vi "Test Config Iface Readback U32.vi"(8 "error in (no error)":errorcluster, 11 "Test Case In":refnum<class "Configuration Interface Test.lvclass">) -> (0 "error out":errorcluster, 3 "Test Case Out":refnum<class "Configuration Interface Test.lvclass">)   [LabVIEW 2020, in "Configuration Interface Test.lvclass"]
uses:
  Configuration Interface Test.lvclass
  C:/Program Files (x86)/National Instruments/LabVIEW 2020/vi.lib/Asteme/LUnit/Test Case.lvclass
  Framework/Configuration/Configuration.lvclass
  <vilib>/Asteme/LUnit/Test Case.lvclass/Test Case.ctl
  <vilib>/Asteme/LUnit/LUnit Assertion Result.lvclass/LUnit Assertion Result.ctl
  <vilib>/Asteme/LUnit/Palette/Pass.vi
  <vilib>/Asteme/LUnit/Palette/Fail.vi
  <vilib>/Asteme/LUnit/Variant to string.vi
  <vilib>/Asteme/LUnit/Set Assertion Type.vi
  <vilib>/Asteme/LUnit/Add test result.vi
  <vilib>/Asteme/LUnit/LUnit Get Test Case.vi
  <vilib>/Asteme/LUnit/Assertion Result/LUnit Get Test Name.vi
  <vilib>/Asteme/LUnit/LUnit Write Message.vi
  <vilib>/Asteme/LUnit/LUnit Write Description.vi
  <vilib>/Asteme/LUnit/LUnit Write Skipped.vi
  <vilib>/Asteme/LUnit/LUnit Write Passed.vi
  <vilib>/Asteme/LUnit/LUnit Write Assertion Type.vi
  <vilib>/Asteme/LUnit/Read Test Case Name.vi
  <vilib>/Utility/Data Type/Get Type Information.vi
  <vilib>/Utility/LVClass/Get LV Class Name.vi
  <vilib>/Asteme/LUnit/LUnit Assertion Result.lvclass
  <vilib>/Asteme/LUnit/Test Case.lvclass
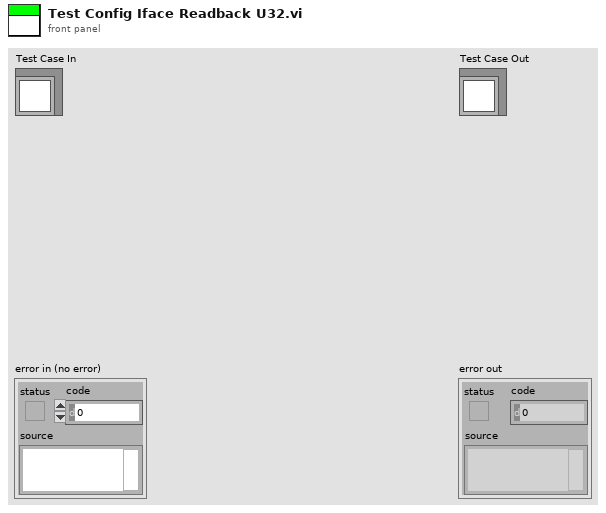
[diagram p1: front panel]
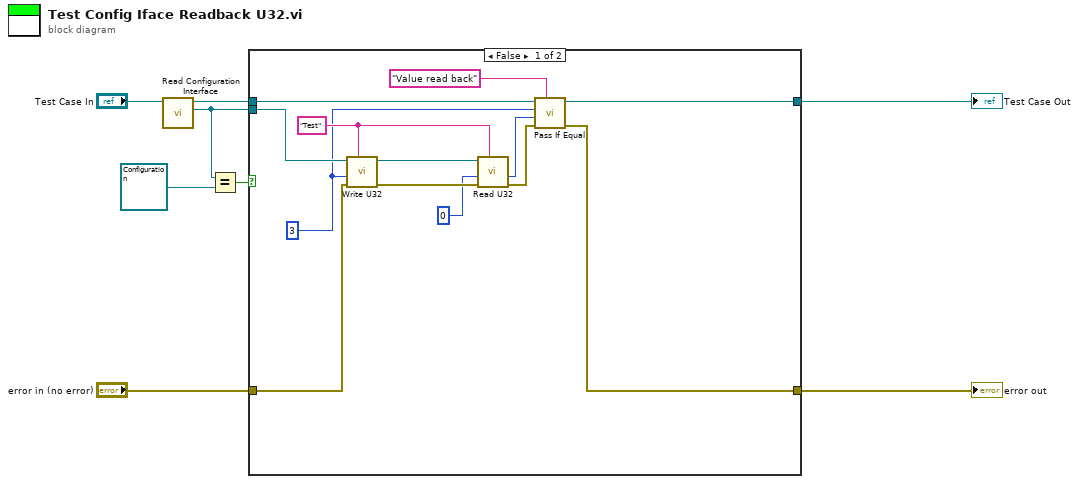
[diagram p0: block diagram]
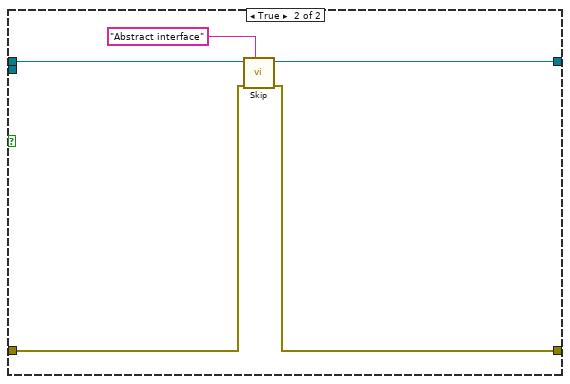
[diagram p2: hidden frame]
diagram:
  n1 = call "Read Configuration Interface.vi"("Configuration Interface Test In"="Test Case In") -> ("Configuration"=w3:refnum<class "Configuration.lvclass">, "Configuration Interface Test Out"=w6:refnum<class "Configuration Interface Test.lvclass">)  [unwired: 9 in]
  n2 = Equal?(x=w3, y=refnum<class "Configuration.lvclass"> refnum ("Configuration")) -> (x = y?=w1:bool)
  n3 = case shown="False" w1 {
    tunnel: [w18 w23] -> w7
    tunnel: w6 -> [w17 w26]
    tunnel: [w16 w25] -> w5
    tunnel: "error in (no error)" -> [w11 w24]
    tunnel: w3 -> [w14 _]
    frame False {
      w10 = u32 3
      w19 = "Test" ("key")
      n4 = call-dynamic "Write U32.vi"("key"=w19, "error in (no error)"=w11, "Value"=w10, "Configuration File In"=w14) -> ("error out"=w20:errorcluster, "Configuration File Out"=w21:refnum<class "Configuration.lvclass">)  [unwired: 6 in]
      n5 = call-dynamic "Read U32.vi"("key"=w19, "error in (no error)"=w20, "default value"=u32 0, "Configuration File In"=w21) -> ("error out"=w15:errorcluster, "value"=w12:u32)  [unwired: 5 in, 1 out]
      n6 = call <vilib>:"Pass If Equal.vi"("Description"="Value read back", "error in (no error)"=w15, "Actual"=w12, "Expected"=w10, "Test Case In"=w17) -> ("error out"=w18:errorcluster, "Test Case Out"=w16:refnum<class "Configuration Interface Test.lvclass">)  [unwired: 5 in]
    }
    frame True {
      n7 = call <vilib>:"Skip.vi"("Description"="Abstract interface", "error in (no error)"=w24, "Test Case In"=w26) -> ("error out"=w23:errorcluster, "Test Case Out"=w25:refnum<class "Configuration Interface Test.lvclass">)  [unwired: 7 in]
    }
  }
  "error out" <- w7
  "Test Case Out" <- w5
